vi "validate configuration.vi"(8 "error in":errorcluster, 11 "UI Reference configuration in":refnum<class "UI Reference configuration.lvclass">) -> (0 "error out":errorcluster, 3 "UI Reference configuration out":refnum<class "UI Reference configuration.lvclass">)   [LabVIEW 2013, in "UI Reference configuration.lvclass"]
doc: "This function performs validation of the configuration. This function should be safe to call at any point and should not rely on anything in the runtime environment."
uses:
  UI Reference configuration.lvclass
  <vilib>/NI/Tag Bus Module Framework/module configuration/TBM module configuration.lvclass
  UI Reference configuration.lvclass/UI Reference configuration.ctl
  Read VI name.vi
  Read VI Refnum.vi
  <vilib>/NI/Tag Bus Module Framework/root configuration/TBM configuration.lvclass
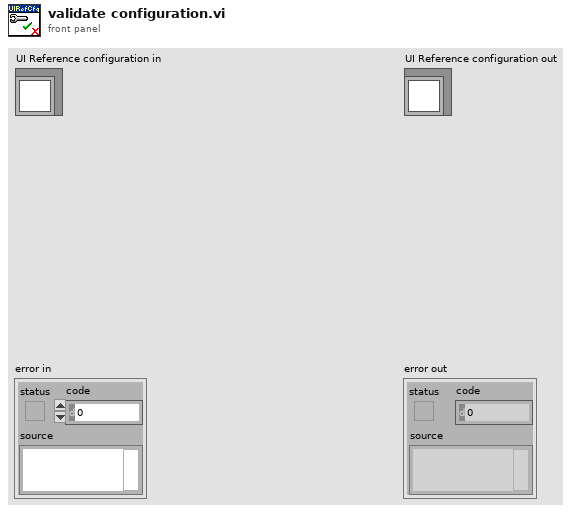
[diagram p1: front panel]
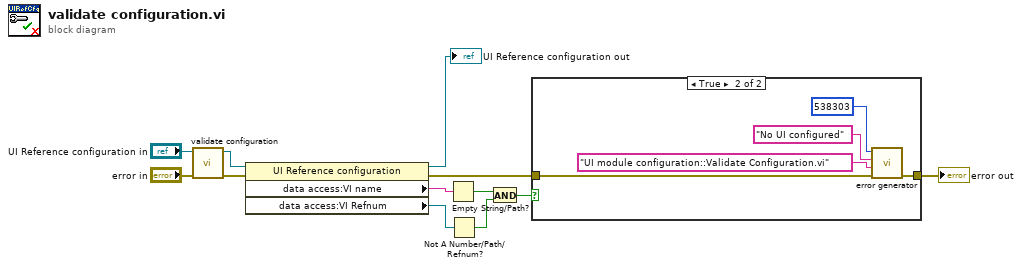
[diagram p0: block diagram]
diagram:
  n1 = call-parent "validate configuration.vi"("error in"="error in", "configuration in"="UI Reference configuration in") -> ("error out"=w12:errorcluster, "configuration out"=w9:refnum<class "UI Reference configuration.lvclass">)  [unwired: 8 in]
  n2 = property class="UI Reference configuration"(reference=w9, error in=w12) -> (reference out=→"UI Reference configuration out":refnum<class "UI Reference configuration.lvclass">, error out=w7:errorcluster, "data access:VI name"=w5:string, "data access:VI Refnum"=w4:refnum<vi>)
  n3 = Empty String/Path?(string/path=w5) -> (empty?=w2:bool)
  n4 = Not A Number/Path/Refnum?(number/path/refnum=w4) -> (NaN/Path/Refnum?=w3:bool)
  n5 = And(x=w2, y=w3) -> (x .and. y?=w1:bool)
  n6 = case shown="True" w1 {
    tunnel: w7 -> [w13 w15]
    tunnel: [w13 w14] -> w6
    frame False {
    }
    frame True {
      n7 = call <vilib>:"error generator.vi"("error in"=w15, "source"="UI module configuration::Validate Configuration.vi", "append error message"="No UI configured", "error code (0)"=538303) -> ("error out"=w14:errorcluster)  [unwired: 7 in]
    }
  }
  "error out" <- w6
